vi "Teleop.vi"(10 "Match Info":T1={"Autonomous Elapsed Seconds"=0.0, "TeleOp Elapsed Seconds"=0.0, "Disabled Elapsed Seconds"=0.0, "Visited Autonomous"=FALSE, "Visited TeleOp"=FALSE, "Visited Disabled"=FALSE, "Autonomous Settings"={"Autonomous Style"=enum."Independent", "VI Refnum"=refnum}}, 11 "Call Context":T2) -> ()   [LabVIEW 2013]
doc: "This VI is called for each TeleOp packet received from the DS where the robot is not disabled. It is often used to read from the joysticks and update I/O or to update setpoints for timed control loops. It should complete and return within 20 milliseconds or it may miss DS packets."
uses:
  <vilib>/Rock Robotics/WPI/DriverStation/WPI_DriverStationDerivedRobotMode.ctl
  <vilib>/Rock Robotics/WPI/DriverStation/WPI_DriverStationMatch Info.ctl
  <vilib>/Rock Robotics/WPI/Solenoid/WPI_SolenoidValue.ctl
  Robot Global Data.vi
  <vilib>/Rock Robotics/WPI/Joystick/WPI_JoystickGetSetRefNum.vi
  <vilib>/Rock Robotics/WPI/RobotDrive/WPI_RobotDriveGetSetRefNum.vi
  <vilib>/Rock Robotics/WPI/Solenoid/WPI_SolenoidSetEnum.vi
  <vilib>/Rock Robotics/WPI/Solenoid/Deprecated/WPI_SolenoidGetBool.vi
  Labview/Sub VIs/Sting Pot Value.vi
panel:
  out "Voltage":dbl
  out "Value":bool
  out "Numeric 1":dbl(slide) scale=0.0..100.0
  out "Boolean 2":bool
  out "Boolean 1":bool
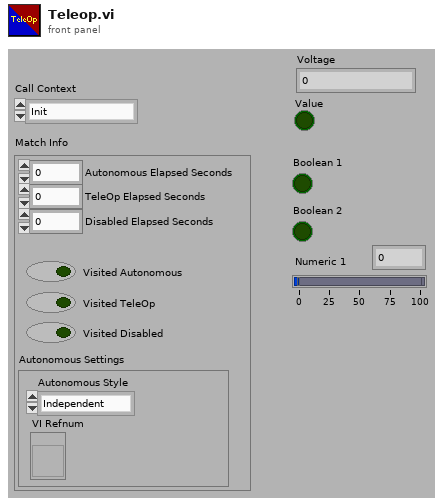
[diagram p1: front panel]
types:
  T1 = typedef "WPI_DriverStationMatch Info.ctl" = cluster{"Autonomous Elapsed Seconds":dbl, "TeleOp Elapsed Seconds":dbl, "Disabled Elapsed Seconds":dbl, "Visited Autonomous":bool, "Visited TeleOp":bool, "Visited Disabled":bool, "Autonomous Settings":cluster{"Autonomous Style":enum16{"Iterative", "Independent"}, "VI Refnum":refnum<vi>}}
  T2 = typedef "WPI_DriverStationDerivedRobotMode.ctl" = enum16{"Init", "Execute", "Stop"}
  T3 = typedef "WPI_JoystickDevRef.ctl" = cluster{"Device":T4}
  T4 = typedef "WPI_JoystickDeviceEnum.ctl" = enum16{"USB 1", "USB 2", "USB 3", "USB 4", "Kinect 1", "Kinect 2"}
  T5 = typedef "WPI_AnalogChannelDevRef.ctl" = cluster{"DevStatus":errorcluster, "Analog Module":T6, "Analog Channel":T7}
  T6 = typedef "FPGA_TypedefAnalogModule.ctl" = enum16{"Analog Module 1", "Analog Module 2"}
  T7 = typedef "FPGA_AIChannel.ctl" = enum8{"AI 1", "AI 2", "AI 3", "AI 4", "AI 5", "AI 6", "AI 7", "AI 8", "Invalid"}
  T8 = typedef "WPI_JoystickButtonState.ctl" = cluster{"Button 1":bool, "Button 2":bool, "Button 3":bool, "Button 4":bool, "Button 5":bool, "Button 6":bool, "Button 7":bool, "Button 8":bool, "Button 9":bool, "Button 10":bool, "Button 11":bool, "Button 12":bool}
  T9 = cluster{"axis 1 (x)":dbl, "axis 2 (y)":dbl, "axis 3 (throttle)":dbl, "axis 4":dbl, "axis 5":dbl, "axis 6":dbl}
  T10 = typedef "WPI_RobotDriveDevRef.ctl" = cluster{"DevStatus":errorcluster, "Motors[]":T11[], "Square Inputs":bool, "Max Output":dbl, "Isochronous":bool}
  T11 = typedef "WPI_MotorControlDeviceRef.ctl" = cluster{"DeviceStatus":errorcluster, "Type":enum16{"PWM", "CAN"}, "PWM":cluster{"Digital Module":T12, "PWM Channel":T13, "DeadBand":T14}, "CAN":cluster{"Device Number":u8, "Control Mode":T15, "Semaphore":T16, "Max Vout":dbl}, "Invert":bool, "TransformRef":T17, "InvTransformRef":T17}
  T12 = typedef "FPGA_TypedefDigitalModule.ctl" = enum16{"Digital Module 1", "Digital Module 2"}
  T13 = typedef "FPGA_DIOPWMChannel.ctl" = enum8{"PWM 1", "PWM 2", "PWM 3", "PWM 4", "PWM 5", "PWM 6", "PWM 7", "PWM 8", "PWM 9", "PWM 10", "Invalid"}
  T14 = typedef "WPI_PWMDeadband.ctl" = cluster{"Name":string, "maxPositivePwm":i32, "minPositivePwm":i32, "centerPwm":i32, "maxNegativePwm":i32, "minNegativePwm":i32, "angularRange":u16}
  T15 = typedef "WPI_CANJaguar_ControlMode.ctl" = enum8{"Percent VBus", "Current", "Speed", "Position", "Voltage"}
  T16 = typedef "Semaphore RefNum" = refnum<k1>
  T17 = typedef "WPI_PWMTransform_ConPane.ctl" = refnum<vi>
  T18 = typedef "WPI_RelayDevRef.ctl" = cluster{"DevStatus":errorcluster, "Relay Channel":T19, "Digital Module":T12, "Relay Direction":T20}
  T19 = typedef "FPGA_DIORelayChannel.ctl" = enum8{"Relay 1", "Relay 2", "Relay 3", "Relay 4", "Relay 5", "Relay 6", "Relay 7", "Relay 8", "Invalid"}
  T20 = typedef "WPI_RelayDirection.ctl" = enum16{"Both directions", "Forward only", "Reverse only"}
  T21 = typedef "WPI_DigitalInputDevRef.ctl" = cluster{"DevStatus":errorcluster, "DIO Channel":T22, "Digital Module":T12}
  T22 = typedef "FPGA_DIOChannel.ctl" = enum8{"DIO 1", "DIO 2", "DIO 3", "DIO 4", "DIO 5", "DIO 6", "DIO 7", "DIO 8", "DIO 9", "DIO 10", "DIO 11", "DIO 12", "DIO 13", "DIO 14", "Invalid"}
  T23 = typedef "WPI_SolenoidDevRef.ctl" = cluster{"DevStatus":errorcluster, "Solenoid Module":T24, "Forward Solenoid Channel":T25, "Reverse Solenoid Channel":T25}
  T24 = typedef "FPGA_TypedefSolenoidModule.ctl" = enum16{"Solenoid Module 1", "Solenoid Module 2"}
  T25 = typedef "WPI_SolenoidChannel.ctl" = enum8{"Solenoid 1", "Solenoid 2", "Solenoid 3", "Solenoid 4", "Solenoid 5", "Solenoid 6", "Solenoid 7", "Solenoid 8", "Invalid"}
  T26 = typedef "WPI_SolenoidValue.ctl" = enum16{"Off", "On", "Forward", "Reverse"}
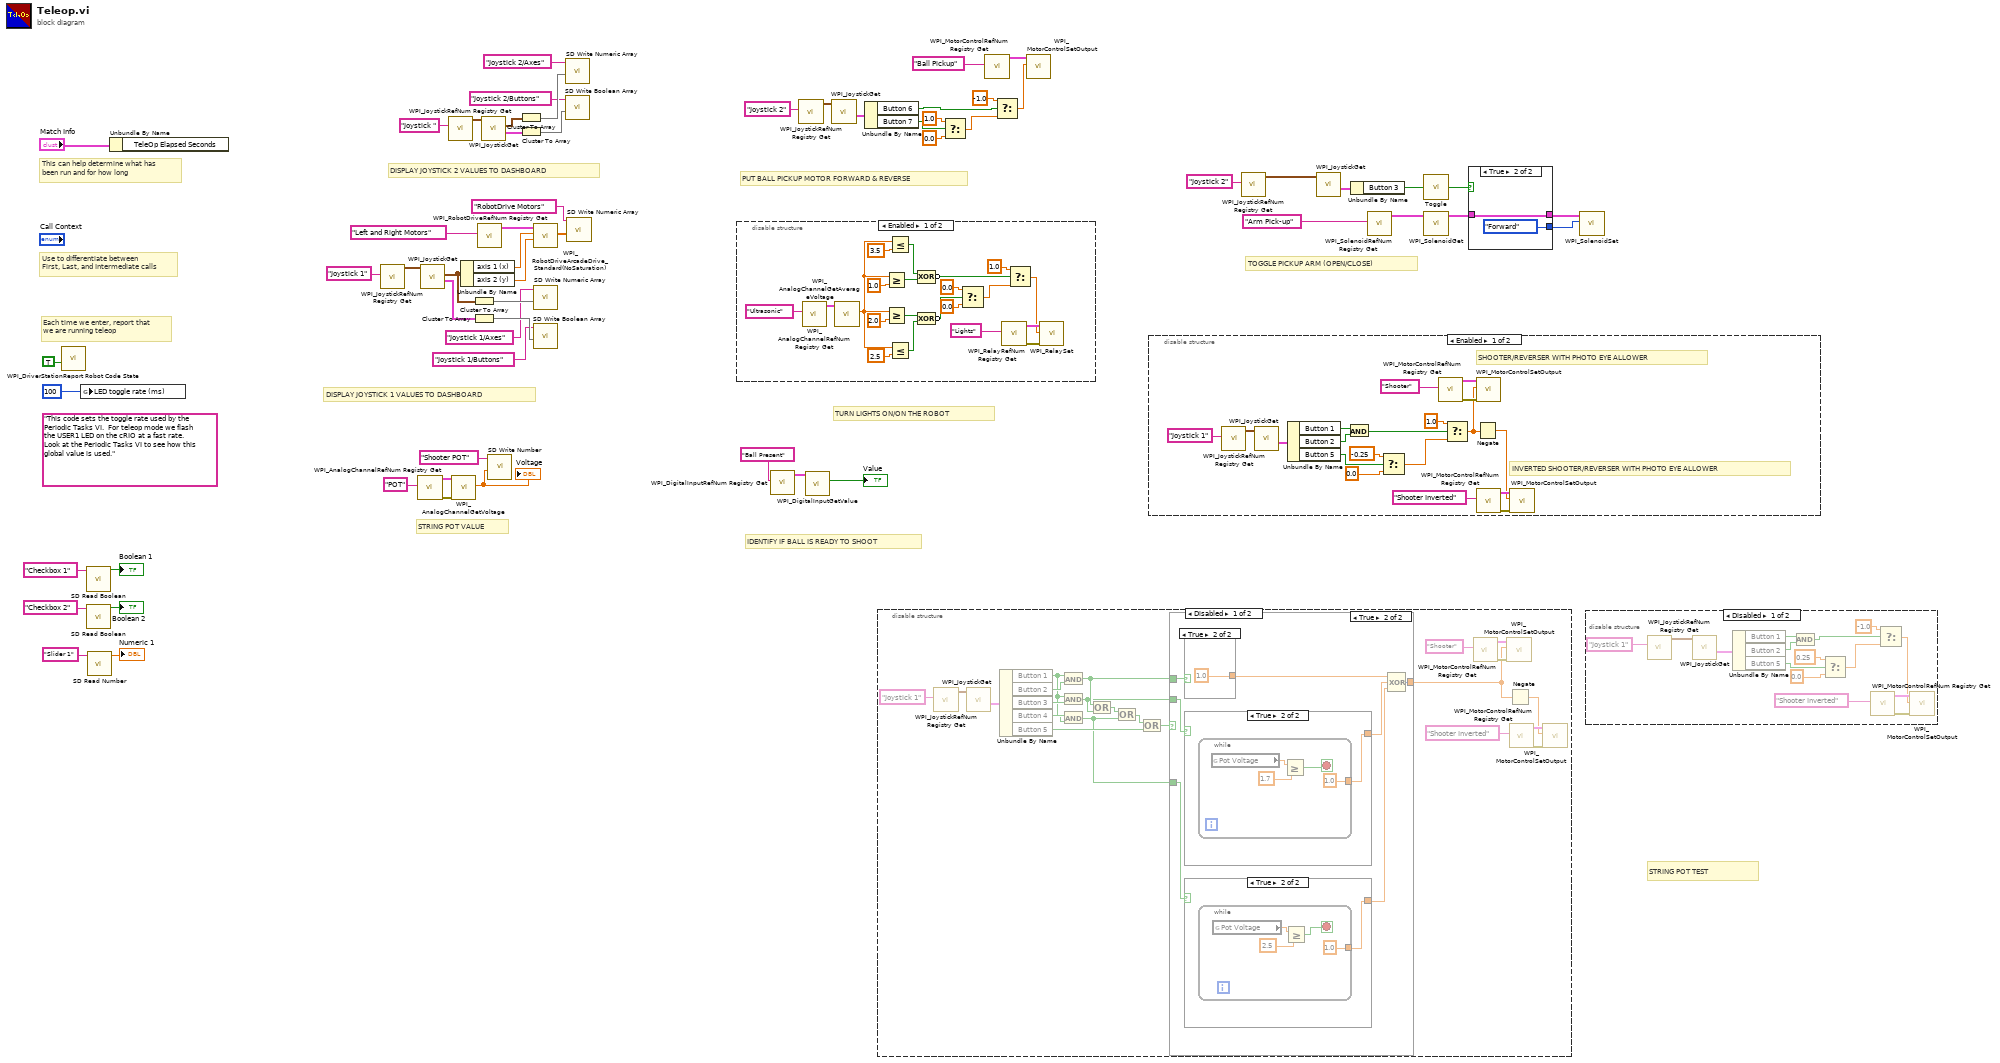
[diagram p0: block diagram]
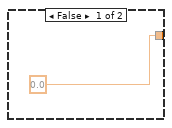
[diagram p2: hidden frame]
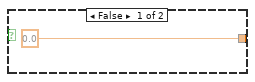
[diagram p3: hidden frame]
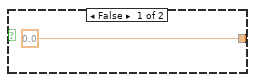
[diagram p4: hidden frame]
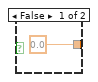
[diagram p5: hidden frame]
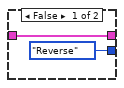
[diagram p10: hidden frame]
diagram:
  (unwired) "This code sets the toggle rate used by the Periodic Tasks VI.  For teleop mode we flash the USER1 LED on the cRIO at a fast rate.  Look at the Periodic Tasks VI to see how this global value is used."
  # "STRING POT TEST"
  # "TOGGLE PICKUP ARM (OPEN/CLOSE)"
  # "PUT BALL PICKUP MOTOR FORWARD & REVERSE"
  # "DISPLAY JOYSTICK 1 VALUES TO DASHBOARD"
  # "DISPLAY JOYSTICK 2 VALUES TO DASHBOARD"
  # "IDENTIFY IF BALL IS READY TO SHOOT"
  # "TURN LIGHTS ON/ON THE ROBOT"
  # "STRING POT VALUE"
  # "Each time we enter, report that\nwe are running teleop"
  # "Use to differentiate between\nFirst, Last, and Intermediate calls"
  # "This can help determine what has\nbeen run and for how long"
  n1 = call <vilib>:"WPI_DriverStationReport Robot Code State.vi"("TeleOp"=TRUE ("Autonomous")) -> ()  [unwired: 10 in, 1 out]
  n2 = global write "Robot Global Data.vi" "LED toggle rate (ms)"(u32 100 ("LED ms toggle rate")) -> ()
  n3 = call <vilib>:"SD Read Boolean.vi"("Name"="Checkbox 1" ("refnum name")) -> ("Boolean"=→"Boolean 1":bool)  [unwired: 8 in, 2 out]
  n4 = call <vilib>:"SD Read Boolean.vi"("Name"="Checkbox 2" ("refnum name")) -> ("Boolean"=→"Boolean 2":bool)  [unwired: 8 in, 2 out]
  n5 = call <vilib>:"SD Read Number.vi"("Name"="Slider 1" ("refnum name")) -> ("Numeric"=→"Numeric 1":dbl)  [unwired: 8 in, 2 out]
  n6 = Unbundle By Name("Match Info") -> ()  [unwired: 1 out]
  n7 = call <vilib>:"WPI_JoystickRefNum Registry Get.vi"("refnum name"="Joystick 1") -> ("JoystickDevRef"=w55:T3)  [unwired: 1 in, 9 out]
  n8 = call <vilib>:"WPI_AnalogChannelRefNum Registry Get.vi"("refnum name"="POT") -> ("error out"=w17:errorcluster, "AIDeviceRef"=w18:T5)  [unwired: 9 in]
  n9 = call <vilib>:"WPI_JoystickGet.vi"("JoystickDevRef"=w55) -> ("Buttons"=w52:T8, "Axes"=w49:T9)  [unwired: 1 in, 4 out]
  n10 = call <vilib>:"WPI_JoystickRefNum Registry Get.vi"("refnum name"="Joystick ") -> ("JoystickDevRef"=w7:T3)  [unwired: 1 in, 9 out]
  n11 = call <vilib>:"WPI_AnalogChannelGetVoltage.vi"("error in (no error)"=w17, "AIDeviceRef"=w18) -> ("Voltage"=w15:dbl)  [unwired: 7 in, 2 out]
  "Voltage" <- w15
  n12 = Unbundle By Name(w49) -> ("axis 1 (x)"=w58:dbl, "axis 2 (y)"=w57:dbl)
  n13 = Cluster To Array(cluster=w49) -> (array=w48:dbl[])
  n14 = Cluster To Array(cluster=w52) -> (array=w51:bool[])
  n15 = call <vilib>:"WPI_RobotDriveRefNum Registry Get.vi"("refnum name"="Left and Right Motors") -> ("RobotDriveDevRef"=w59:T10)  [unwired: 1 in, 9 out]
  n16 = call <vilib>:"WPI_JoystickGet.vi"("JoystickDevRef"=w7) -> ("Buttons"=w8:T8, "Axes"=w11:T9)  [unwired: 1 in, 4 out]
  n17 = call <vilib>:"SD Write Number.vi"("Numeric"=w15, "Name"="Shooter POT" ("Table Prefix out")) -> ()  [unwired: 8 in, 2 out]
  n18 = Cluster To Array(cluster=w11) -> (array=w12:dbl[])
  n19 = Cluster To Array(cluster=w8) -> (array=w9:bool[])
  n20 = call <vilib>:"WPI_RobotDriveArcadeDrive_Standard(NoSaturation).vi"("Y axis value"=w57, "X axis value"=w58, "RobotDriveDevRef"=w59) -> ("Motor Values"=w45:dbl[])  [unwired: 1 in, 7 out]
  n21 = call <vilib>:"SD Write Numeric Array.vi"("Numeric Array"=w48, "Name"="Joystick 1/Axes") -> ()  [unwired: 8 in, 2 out]
  n22 = call <vilib>:"SD Write Boolean Array.vi"("Boolean Array"=w51, "Name"="Joystick 1/Buttons") -> ()  [unwired: 8 in, 2 out]
  n23 = call <vilib>:"SD Write Numeric Array.vi"("Numeric Array"=w12, "Name"="Joystick 2/Axes") -> ()  [unwired: 8 in, 2 out]
  n24 = call <vilib>:"SD Write Boolean Array.vi"("Boolean Array"=w9, "Name"="Joystick 2/Buttons") -> ()  [unwired: 8 in, 2 out]
  n25 = call <vilib>:"SD Write Numeric Array.vi"("Numeric Array"=w45, "Name"="RobotDrive Motors") -> ()  [unwired: 8 in, 2 out]
  n26 = disable-structure shown="Enabled" {
    frame Enabled {
      n27 = call <vilib>:"WPI_AnalogChannelRefNum Registry Get.vi"("refnum name"="Ultrasonic") -> ("AIDeviceRef"=w81:T5)  [unwired: 9 in, 1 out]
      n28 = call <vilib>:"WPI_AnalogChannelGetAverageVoltage.vi"("AIDeviceRef"=w81) -> ("Voltage"=w72:dbl)  [unwired: 8 in, 2 out]
      n29 = Greater Or Equal?(x=w72, y=1.0) -> (x >= y?=w75:bool)
      n30 = Greater Or Equal?(x=w72, y=2.0) -> (x >= y?=w69:bool)
      n31 = Less Or Equal?(x=w72, y=3.5) -> (x <= y?=w74:bool)
      n32 = Less Or Equal?(x=w72, y=2.5) -> (x <= y?=w70:bool)
      n33 = Compound Arithmetic op=XOR(w74, w75) -> (invert w67:bool)
      n34 = Compound Arithmetic op=XOR(w69, w70) -> (invert w68:bool)
      n35 = Select(t=0.0, s=w68, f=0.0) -> (s? t:f=w63:dbl)
      n36 = call <vilib>:"WPI_RelayRefNum Registry Get.vi"("refnum name"="Lights") -> ("error out"=w80:errorcluster, "RelayDevRef"=w79:T18)  [unwired: 9 in]
      n37 = Select(t=1.0, s=w67, f=w63) -> (s? t:f=w62:dbl)
      n38 = call <vilib>:"WPI_RelaySet.vi"("error in (no error)"=w80, "RelayValue"=w62, "RelayDevRef"=w79) -> ()  [unwired: 7 in, 2 out]
    }
    frame Disabled {
    }
  }
  n39 = call <vilib>:"WPI_DigitalInputRefNum Registry Get.vi"("refnum name"="Ball Present") -> ("DigitalInputDevRef"=w4:T21)  [unwired: 9 in, 1 out]
  n40 = call <vilib>:"WPI_JoystickRefNum Registry Get.vi"("refnum name"="Joystick 2") -> ("JoystickDevRef"=w31:T3)  [unwired: 9 in, 1 out]
  n41 = call <vilib>:"WPI_DigitalInputGetValue.vi"("DigitalInputDevRef"=w4) -> ("Value"=→"Value":bool)  [unwired: 8 in, 2 out]
  n42 = call <vilib>:"WPI_JoystickGet.vi"("JoystickDevRef"=w31) -> ("Buttons"=w32:T8)  [unwired: 4 in, 2 out]
  n43 = Unbundle By Name(w32) -> ("Button 6"=w33:bool, "Button 7"=w29:bool)
  n44 = disable-structure shown="Disabled" {
    frame Disabled {
      n45 = call <vilib>:"WPI_JoystickRefNum Registry Get.vi"("refnum name"="Joystick 1") -> ("JoystickDevRef"=w103:T3)  [unwired: 9 in, 1 out]
      n46 = call <vilib>:"WPI_JoystickGet.vi"("JoystickDevRef"=w103) -> ("Buttons"=w104:T8)  [unwired: 4 in, 2 out]
      n47 = Unbundle By Name(w104) -> ("Button 1"=w99:bool, "Button 2"=w101:bool, "Button 3"=w100:bool, "Button 4"=w98:bool, "Button 5"=w95:bool)
      n48 = And(x=w99, y=w101) -> (x .and. y?=w93:bool)
      n49 = And(x=w99, y=w100) -> (x .and. y?=w92:bool)
      n50 = And(x=w99, y=w98) -> (x .and. y?=w83:bool)
      n51 = Or(x=w93, y=w92) -> (x .or. y?=w97:bool)
      n52 = Or(x=w97, y=w83) -> (x .or. y?=w96:bool)
      n53 = Or(x=w96, y=w95) -> (x .or. y?=w94:bool)
      n54 = case shown="True" w94 {
        tunnel: w93 -> [_ w112]
        tunnel: w92 -> [_ w111]
        tunnel: [0.0 w107] -> w85
        tunnel: w83 -> [_ w106]
        frame False {
        }
        frame True {
          n55 = case shown="True" w112 {
            tunnel: [0.0 1.0] -> w110
            frame False {
            }
            frame True {
            }
          }
          n56 = case shown="True" w111 {
            tunnel: [0.0 w120] -> w109
            frame False {
            }
            frame True {
              n57 = while {
                tunnel: [1.0] -> w120
                stop <- w123 stop-if-true
                n58 = global read "Sting Pot Value.vi" "Pot Voltage"() -> (w122:dbl)
                n59 = Greater Or Equal?(x=w122, y=1.7) -> (x >= y?=w123:bool)
              }
            }
          }
          n60 = case shown="True" w106 {
            tunnel: [0.0 w114] -> w108
            frame False {
            }
            frame True {
              n61 = while {
                tunnel: [1.0] -> w114
                stop <- w115 stop-if-true
                n62 = global read "Sting Pot Value.vi" "Pot Voltage"() -> (w116:dbl)
                n63 = Greater Or Equal?(x=w116, y=2.5) -> (x >= y?=w115:bool)
              }
            }
          }
          n64 = Compound Arithmetic op=XOR(w110, w109, w108) -> (w107:i32)
        }
      }
      n65 = call <vilib>:"WPI_MotorControlRefNum Registry Get.vi"("refnum name"="Shooter") -> ("error out"=w87:errorcluster, "MotorControlDevRef"=w86:T11)  [unwired: 9 in]
      n66 = call <vilib>:"WPI_MotorControlSetOutput.vi"("error in (no error)"=w87, "Output"=w85, "MotorControlDevRef"=w86) -> ()  [unwired: 6 in, 3 out]
      n67 = Negate(x=w85) -> (-x=w84:dbl)
      n68 = call <vilib>:"WPI_MotorControlRefNum Registry Get.vi"("refnum name"="Shooter Inverted") -> ("error out"=w90:errorcluster, "MotorControlDevRef"=w91:T11)  [unwired: 9 in]
      n69 = call <vilib>:"WPI_MotorControlSetOutput.vi"("error in (no error)"=w90, "Output"=w84, "MotorControlDevRef"=w91) -> ()  [unwired: 6 in, 3 out]
    }
    frame Enabled {
    }
  }
  n70 = Select(t=1.0, s=w29, f=0.0) -> (s? t:f=w2:dbl)
  n71 = call <vilib>:"WPI_MotorControlRefNum Registry Get.vi"("refnum name"="Ball Pickup") -> ("MotorControlDevRef"=w37:T11)  [unwired: 9 in, 1 out]
  n72 = Select(t=-1.0, s=w33, f=w2) -> (s? t:f=w1:dbl)
  n73 = call <vilib>:"WPI_MotorControlSetOutput.vi"("Output"=w1, "MotorControlDevRef"=w37) -> ()  [unwired: 7 in, 3 out]
  n74 = disable-structure shown="Enabled" {
    frame Enabled {
      # "SHOOTER/REVERSER WITH PHOTO EYE ALLOWER"
      # "INVERTED SHOOTER/REVERSER WITH PHOTO EYE ALLOWER"
      n75 = call <vilib>:"WPI_JoystickRefNum Registry Get.vi"("refnum name"="Joystick 1") -> ("JoystickDevRef"=w144:T3)  [unwired: 9 in, 1 out]
      n76 = call <vilib>:"WPI_JoystickGet.vi"("JoystickDevRef"=w144) -> ("Buttons"=w143:T8)  [unwired: 4 in, 2 out]
      n77 = Unbundle By Name(w143) -> ("Button 1"=w138:bool, "Button 2"=w139:bool, "Button 5"=w137:bool)
      n78 = And(x=w138, y=w139) -> (x .and. y?=w132:bool)
      n79 = Select(t=-0.25, s=w137, f=0.0) -> (s? t:f=w135:dbl)
      n80 = call <vilib>:"WPI_MotorControlRefNum Registry Get.vi"("refnum name"="Shooter") -> ("error out"=w141:errorcluster, "MotorControlDevRef"=w140:T11)  [unwired: 9 in]
      n81 = Select(t=1.0, s=w132, f=w135) -> (s? t:f=w128:dbl)
      n82 = Negate(x=w128) -> (-x=w127:dbl)
      n83 = call <vilib>:"WPI_MotorControlSetOutput.vi"("error in (no error)"=w141, "Output"=w128, "MotorControlDevRef"=w140) -> ()  [unwired: 6 in, 3 out]
      n84 = call <vilib>:"WPI_MotorControlRefNum Registry Get.vi"("refnum name"="Shooter Inverted") -> ("error out"=w130:errorcluster, "MotorControlDevRef"=w129:T11)  [unwired: 9 in]
      n85 = call <vilib>:"WPI_MotorControlSetOutput.vi"("error in (no error)"=w130, "Output"=w127, "MotorControlDevRef"=w129) -> ()  [unwired: 6 in, 3 out]
    }
    frame Disabled {
    }
  }
  n86 = call <vilib>:"WPI_JoystickRefNum Registry Get.vi"("refnum name"="Joystick 2") -> ("JoystickDevRef"=w26:T3)  [unwired: 9 in, 1 out]
  n87 = call <vilib>:"WPI_JoystickGet.vi"("JoystickDevRef"=w26) -> ("Buttons"=w25:T8)  [unwired: 4 in, 2 out]
  n88 = Unbundle By Name(w25) -> ("Button 3"=w19:bool)
  n89 = call <vilib>:"WPI_SolenoidRefNum Registry Get.vi"("refnum name"="Arm Pick-up") -> ("SolenoidDevRef"=w24:T23)  [unwired: 9 in, 1 out]
  n90 = call "Toggle.vi"("Input"=w19) -> ("Toggled Output"=w23:bool)
  n91 = call-poly <vilib>:"WPI_SolenoidGet.vi"("SolenoidDevRef"=w24) -> ("SolenoidDevRef"=w22:T23)  [unwired: 8 in, 2 out]
  n92 = case shown="True" w23 {
    tunnel: w22 -> [w147 w149]
    tunnel: [w147 w149] -> w21
    tunnel: [WPI_SolenoidValue."Reverse" ("Value") WPI_SolenoidValue."Forward" ("Value")] -> w20
    frame False {
    }
    frame True {
    }
  }
  n93 = call-poly <vilib>:"WPI_SolenoidSet.vi"("Value"=w20, "SolenoidDevRef"=w21) -> ()  [unwired: 8 in, 2 out]
  n94 = disable-structure shown="Disabled" {
    frame Disabled {
      n95 = call <vilib>:"WPI_JoystickRefNum Registry Get.vi"("refnum name"="Joystick 1") -> ("JoystickDevRef"=w163:T3)  [unwired: 9 in, 1 out]
      n96 = call <vilib>:"WPI_JoystickGet.vi"("JoystickDevRef"=w163) -> ("Buttons"=w164:T8)  [unwired: 4 in, 2 out]
      n97 = Unbundle By Name(w164) -> ("Button 1"=w160:bool, "Button 2"=w161:bool, "Button 5"=w156:bool)
      n98 = And(x=w160, y=w161) -> (x .and. y?=w150:bool)
      n99 = Select(t=0.25, s=w156, f=0.0) -> (s? t:f=w155:dbl)
      n100 = call <vilib>:"WPI_MotorControlRefNum Registry Get.vi"("refnum name"="Shooter Inverted") -> ("error out"=w158:errorcluster, "MotorControlDevRef"=w159:T11)  [unwired: 9 in]
      n101 = Select(t=-1.0, s=w150, f=w155) -> (s? t:f=w151:dbl)
      n102 = call <vilib>:"WPI_MotorControlSetOutput.vi"("error in (no error)"=w158, "Output"=w151, "MotorControlDevRef"=w159) -> ()  [unwired: 6 in, 3 out]
    }
    frame Enabled {
    }
  }
